vi "Check Control Class.vi"(8 "error in (no error)":errorcluster, 10 "Supported Classes":string, 11 "Ctl Ref":refnum<vi>) -> (0 "error out":errorcluster, 3 "Ctl Ref out":refnum<vi>)   [LabVIEW 2020, in "MacroAssert.lvlib"]
doc: "Checks that the class name of <B>Ctl Ref</B> is in the comma-separated list of <B>Supported Classes</B>, and injects a custom error if it is not."
uses:
  MacroAssert.lvlib
  Custom Errors/Custom Errors.lvlib
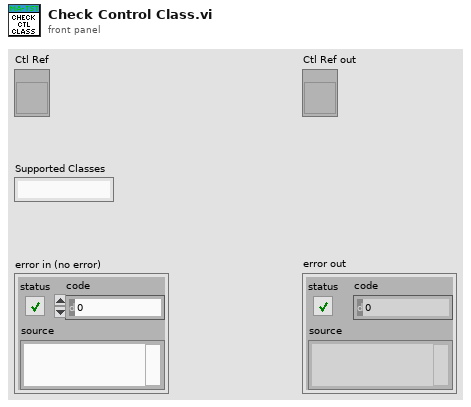
[diagram p1: front panel]
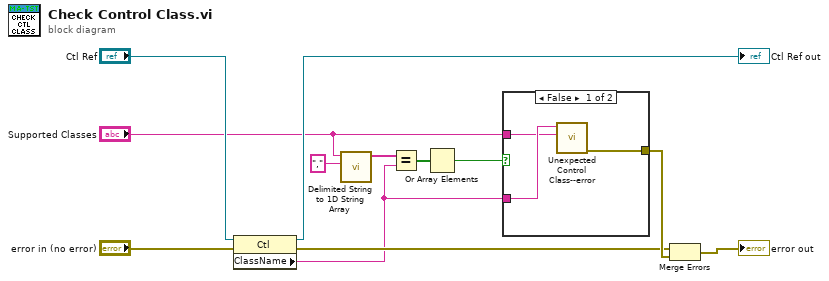
[diagram p0: block diagram]
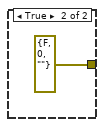
[diagram p2: hidden frame]
diagram:
  n1 = property class="Ctl"(reference="Ctl Ref", error in="error in (no error)") -> (reference out=→"Ctl Ref out":refnum<vi>, error out=w8:errorcluster, "ClassName"=w1:string)
  n2 = call <vilib>:"Delimited String to 1D String Array.vi"("delimiter"=",", "delimited string"="Supported Classes") -> ("string array"=w4:string[])  [unwired: 9 in]
  n3 = Equal?(x=w4, y=w1) -> (x = y?=w3:bool[])
  n4 = Or Array Elements(Boolean array=w3) -> (logical OR=w2:bool)
  n5 = case shown="False" w2 {
    tunnel: "Supported Classes" -> [w13 _]
    tunnel: [w15 errorcluster {"status"=FALSE, "code"=0, "source"=""} ("error out")] -> w11
    tunnel: w1 -> [w14 _]
    frame False {
      n6 = call "Unexpected Control Class--error.vi"("Expected Classes"=w13, "Class Name"=w14) -> ("error out"=w15:errorcluster)  [unwired: 9 in]
    }
    frame True {
    }
  }
  n7 = Merge Errors(w8, w11) -> (→"error out":errorcluster)
